vi "ex7-16.vi"() -> ()   [LabVIEW 2013]
panel:
  out "output cluster":cluster{i32, i32, string, bool}
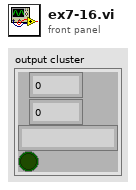
[diagram p1: front panel]
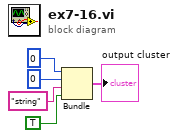
[diagram p0: block diagram]
diagram:
  n1 = Bundle(0, 0, "string", TRUE) -> (→"output cluster":cluster{i32, i32, string, bool})  [unwired: 1 in]
